vi "subvi.vi"(11 "Numeric in":dbl) -> (3 "Numeric out":dbl)   [LabVIEW 2015]
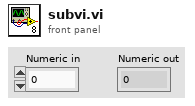
[diagram p1: front panel]
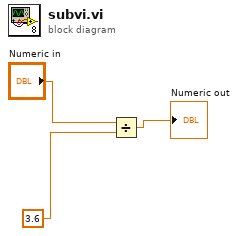
[diagram p0: block diagram]
diagram:
  n1 = Divide(x="Numeric in", y=3.6) -> (x/y=→"Numeric out":dbl)
